vi "ComputeLineROIArray.vi"(7 "ROIDim":T2, 8 "error in (no error)":errorcluster, 10 "ROI In":T1 {"Contours"."Type" items=["No Selection", "Point", "Line", "Rectangle", "Oval", "Polygon", "Freehand Region", "Annulus", "Unused2", "Unused3", "Broken Line", "Freehand Line", "Rotated Rectangle"]}) -> (0 "error out":errorcluster, 2 "ROIArray":T1[](array[typedef]) {"Contours"."Type" items=["No Selection", "Point", "Line", "Rectangle", "Oval", "Polygon", "Freehand Region", "Annulus", "Unused2", "Unused3", "Broken Line", "Freehand Line", "Rotated Rectangle"]})   [LabVIEW 2019]
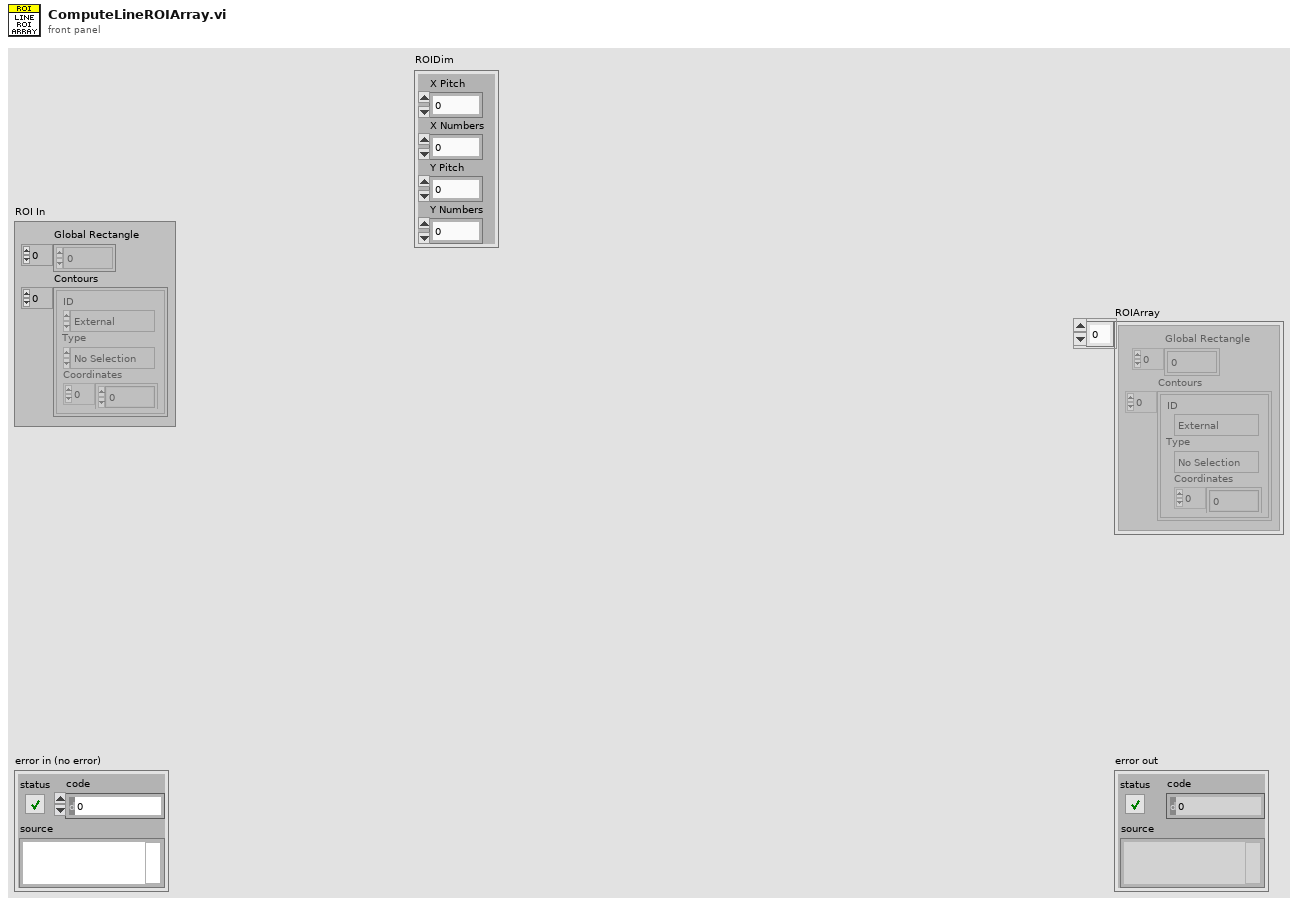
[diagram p1: front panel]
types:
  T1 = typedef "ROI Descriptor" = cluster{"Global Rectangle":i32[], "Contours":cluster{"ID":enum32{"External", "Internal"}, "Type":u32, "Coordinates":i32[]}[]}
  T2 = cluster{"X Pitch":i32, "X Numbers":i32, "Y Pitch":i32, "Y Numbers":i32}
  T3 = typedef "IMAQ Line" = cluster{"Start X":i32, "Start Y":i32, "End X":i32, "End Y":i32}
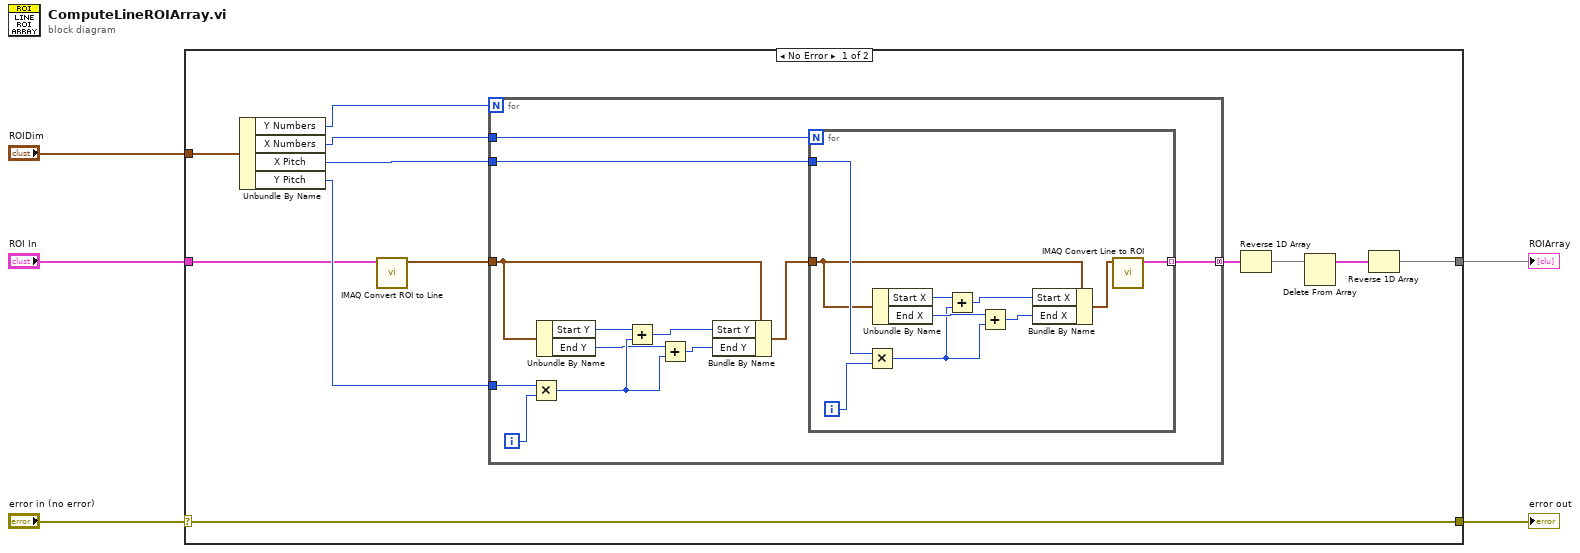
[diagram p0: block diagram]
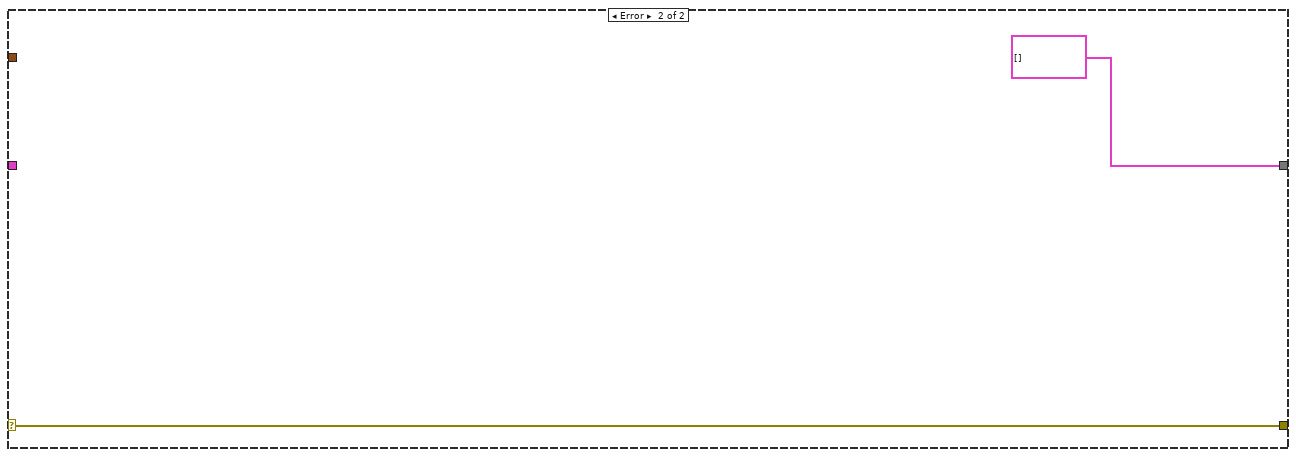
[diagram p2: hidden frame]
diagram:
  n1 = case shown="No Error" "error in (no error)" {
    selector: "error in (no error)" -> [w11 w41]
    tunnel: "ROIDim" -> [w17 _]
    tunnel: [w6 T1[] []] -> w4
    tunnel: [w11 w41] -> w2
    tunnel: "ROI In" -> [w8 _]
    frame No Error {
      n2 = Unbundle By Name(w17) -> ("Y Numbers"=w16:i32, "X Numbers"=w15:i32, "X Pitch"=w13:i32, "Y Pitch"=w14:i32)
      n3 = call "IMAQ Convert ROI to Line"("ROI Descriptor"=w8) -> ("Line"=w9:T3)  [unwired: 8 in, 1 out]
      n4 = for {
        N: w16 -> [_]
        tunnel: w15 -> [w29]
        tunnel: w9 -> [w21]
        tunnel: w14 -> [w22]
        tunnel: w13 -> [w19]
        tunnel: [w18] -> w12 mode=concatenating
        i -> [w23]
        n5 = Multiply(x=w22, y=w23) -> (x*y=w28:i32)
        n6 = Unbundle By Name(w21) -> ("Start Y"=w26:i32, "End Y"=w25:i32)
        n7 = Add(x=w26, y=w28) -> (x+y=w27:i32)
        n8 = Add(x=w25, y=w28) -> (x+y=w24:i32)
        n9 = Bundle By Name(cluster=w21, "Start Y"=w27, "End Y"=w24) -> (w20:T3)
        n10 = for {
          N: w29 -> [_]
          tunnel: w20 -> [w32]
          tunnel: w19 -> [w34]
          tunnel: [w30] -> w18 mode=indexing
          i -> [w31]
          n11 = Multiply(x=w34, y=w31) -> (x*y=w35:i32)
          n12 = Unbundle By Name(w32) -> ("Start X"=w37:i32, "End X"=w38:i32)
          n13 = Add(x=w37, y=w35) -> (x+y=w36:i32)
          n14 = Add(x=w38, y=w35) -> (x+y=w39:i32)
          n15 = Bundle By Name(cluster=w32, "Start X"=w36, "End X"=w39) -> (w33:T3)
          n16 = call "IMAQ Convert Line to ROI"("Line"=w33) -> ("ROI Descriptor"=w30:T1)  [unwired: 8 in, 1 out]
        }
      }
      n17 = Reverse 1D Array(array=w12) -> (reversed array=w7:T1[])
      n18 = Delete From Array(array=w7) -> (array with subset deleted=w10:T1[])  [unwired: 2 in, 1 out]
      n19 = Reverse 1D Array(array=w10) -> (reversed array=w6:T1[])
    }
    frame Error {
    }
  }
  "ROIArray" <- w4
  "error out" <- w2
